vi "Sort By Updated.vi"(10 "Panel B":refnum<class "Panel.lvclass">, 11 "Panel A":refnum<class "Panel.lvclass">) -> (3 "A < B":bool)   [LabVIEW 2020, in "PicoG-App.lvlib" / "AppListPanel.lvclass"]
uses:
  AppListPanel.lvclass
  <vilib>/IlluminatedG/IG OOPanel/OOPanel/Panel/Panel.lvclass
  GWebAppArrayPanel/GWebAppArrayPanel.lvclass
  ViaApp/ViaApp.lvclass
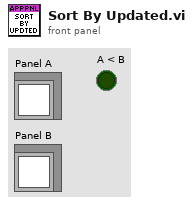
[diagram p1: front panel]
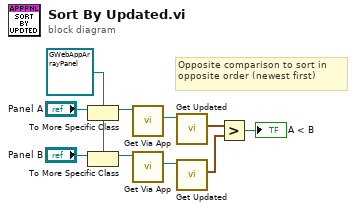
[diagram p0: block diagram]
diagram:
  w8 = refnum<class "GWebAppArrayPanel.lvclass"> refnum ("PicoG-App.lvlib:GWebAppArrayPanel.lvclass")
  # "Opposite comparison to sort in opposite order (newest first)"
  n1 = To More Specific Class(target class=w8, reference="Panel A") -> (specific class reference=w7:refnum<class "GWebAppArrayPanel.lvclass">)  [unwired: 1 in, 1 out]
  n2 = To More Specific Class(target class=w8, reference="Panel B") -> (specific class reference=w6:refnum<class "GWebAppArrayPanel.lvclass">)  [unwired: 1 in, 1 out]
  n3 = call "Get Via App.vi"("GWebAppArrayPanel in"=w7) -> ("App"=w4:refnum<class "ViaApp.lvclass">)  [unwired: 8 in, 2 out]
  n4 = call "Get Via App.vi"("GWebAppArrayPanel in"=w6) -> ("App"=w5:refnum<class "ViaApp.lvclass">)  [unwired: 8 in, 2 out]
  n5 = call "Get Updated.vi"("ViaApp in"=w4) -> ("Last Update"=w3:timestamp)  [unwired: 8 in, 2 out]
  n6 = call "Get Updated.vi"("ViaApp in"=w5) -> ("Last Update"=w2:timestamp)  [unwired: 8 in, 2 out]
  n7 = Greater?(x=w3, y=w2) -> (0:→"A < B":bool)
